vi "Constructor.vi"(8 "error in (no error)":errorcluster) -> (0 "error out":errorcluster, 3 "Collection out":refnum<class "CollectionByValue.lvclass">)   [LabVIEW 2021, in "Collection.lvlib" / "CollectionByValue.lvclass"]
uses:
  CollectionByValue.lvclass
  CollectionByValue.lvclass/CollectionByValue.ctl
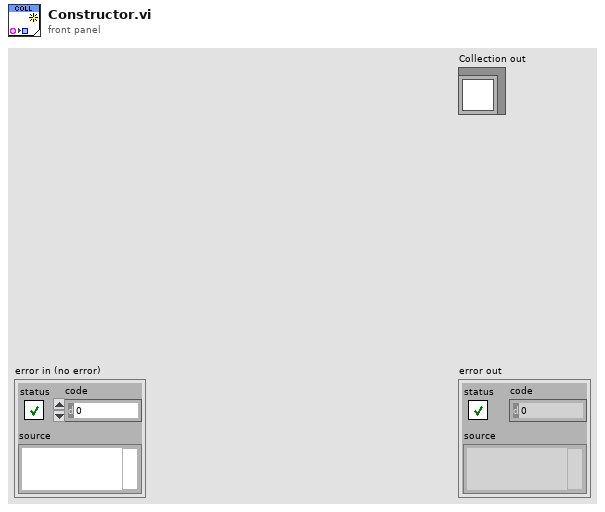
[diagram p1: front panel]
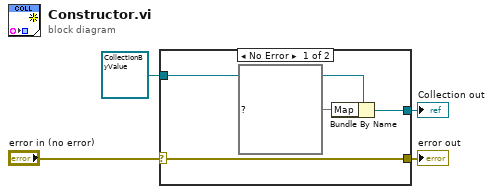
[diagram p0: block diagram]
diagram:
  n1 = case shown="No Error" "error in (no error)" {
    selector: "error in (no error)" -> [w8 w10]
    tunnel: [w8 w10] -> w3
    tunnel: [w6 w9] -> w2
    tunnel: refnum<class "CollectionByValue.lvclass"> refnum ("Collection in") -> [w7 w9]
    frame No Error {
      n2 = Bundle By Name(cluster=w7, "Map"=map{string, refnum<class>} {}) -> (w6:refnum<class "CollectionByValue.lvclass">)
    }
    frame Error {
    }
  }
  "error out" <- w3
  "Collection out" <- w2
